vi "Queue Error Messages.vi"(8 "error in (no error)":errorcluster, 10 "Error Array":T1[](array[typedef]), 11 "queue out":refnum<queue>) -> (0 "error out":errorcluster)   [LabVIEW 2023, in "J1939 Workspace Shared.lvlib"]
uses:
  J1939 Workspace Shared.lvlib
  Addon/Addon Shared/Types/Error Cluster.ctl
  Addon/Addon Shared/Types/Error Types.ctl
  Addon/Addon Shared/J1939 Addon Shared.lvlib
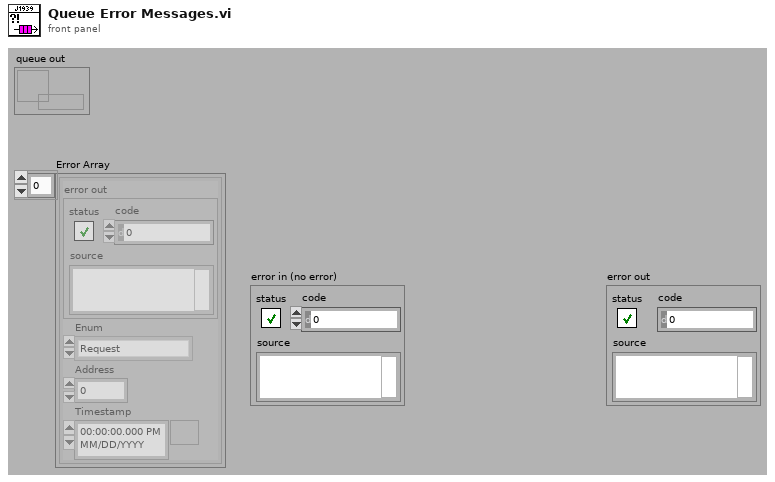
[diagram p1: front panel]
types:
  T1 = typedef "J1939 Addon Shared.lvlib/Error Cluster.ctl" = cluster{"error out":errorcluster, "Enum":T2, "Address":u8, "Timestamp":timestamp}
  T2 = typedef "J1939 Addon Shared.lvlib/Error Types.ctl" = enum16{"Request", "RAW Generation", "Clear Active DTCs", "Clear Previous DTCs", "Addresses", "TLAs", "Get Active DTCs", "Get Previous DTCs", "TCP Connection"}
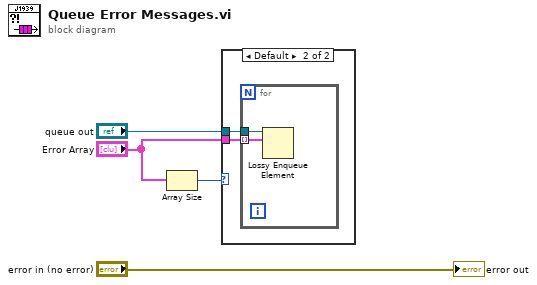
[diagram p0: block diagram]
diagram:
  n1 = Array Size(array="Error Array") -> (size(s)=w1:i32)
  n2 = case shown="Default" w1 {
    tunnel: "queue out" -> [_ w6]
    tunnel: "Error Array" -> [_ w5]
    frame 0 {
    }
    frame Default {
      n3 = for {
        tunnel: w5 -> [w8] mode=indexing
        tunnel: w6 -> [w7]
        n4 = Lossy Enqueue Element(queue=w7, element=w8) -> ()  [unwired: 1 in, 4 out]
      }
    }
  }
  "error out" <- "error in (no error)"
